vi "enqueueMessage.vi"(7 "High Priority (F)":bool, 8 "error in (no error)":errorcluster, 11 "Message":T1) -> (0 "error out":errorcluster)   [LabVIEW 2017, in "loggingModule.lvlib"]
uses:
  loggingModule.lvlib
  TypeDefs/message.ctl
  TypeDefs/queueFGVState.ctl
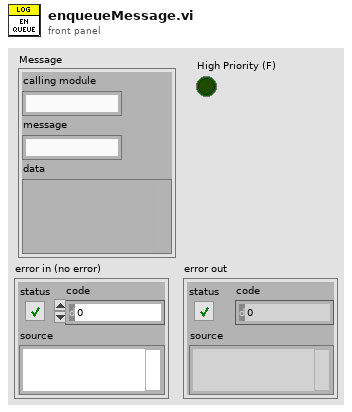
[diagram p1: front panel]
types:
  T1 = typedef "loggingModule.lvlib/message.ctl" = cluster{"calling module":string, "message":string, "data":variant}
  T2 = typedef "loggingModule.lvlib/queueFGVState.ctl" = enum16{"set", "get"}
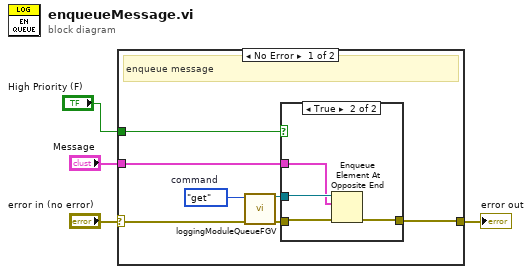
[diagram p0: block diagram]
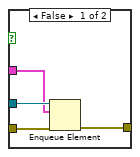
[diagram p2: hidden frame]
diagram:
  n1 = case shown="No Error" "error in (no error)" {
    selector: "error in (no error)" -> [w11 w20]
    tunnel: [w9 w20] -> w3
    tunnel: "Message" -> [w6 _]
    tunnel: "High Priority (F)" -> [w5 _]
    frame No Error {
      w7 = queueFGVState."get"  # command
      # "enqueue message"
      n2 = call "loggingModuleQueueFGV.vi"("error in (no error)"=w11, "command"=w7) -> ("error out"=w10:errorcluster, "queue out"=w8:refnum<queue>)  [unwired: 8 in]
      n3 = case shown="True" w5 {
        tunnel: w10 -> [w15 w19]
        tunnel: [w14 w18] -> w9
        tunnel: w8 -> [w13 w17]
        tunnel: w6 -> [w12 w16]
        frame False {
          n4 = Enqueue Element(queue=w13, element=w12, error in (no error)=w15) -> (error out=w14:errorcluster)  [unwired: 1 in, 2 out]
        }
        frame True {
          n5 = Enqueue Element At Opposite End(queue=w17, element=w16, error in (no error)=w19) -> (error out=w18:errorcluster)  [unwired: 1 in, 2 out]
        }
      }
    }
    frame Error {
    }
  }
  "error out" <- w3
